vi "Send Voltage.vi"(8 "error in":errorcluster, 11 "69X_79X in":refnum<class "6972A.lvclass">) -> (0 "error out":errorcluster, 3 "69X_79X out":refnum<class "6972A.lvclass">)   [LabVIEW 2019, in "6972A.lvlib" / "6972A.lvclass"]
uses:
  Library/6972A.lvclass
  C:/Users/Public/Documents/Development/builds/Instruments/PowerSupply.lvlibp/Library/PowerSupply.lvclass
  Accessors/Read Local Resource.vi
  Accessors/Write Local Resource.vi
  <instrlib>/Agilent N6900 N7900 Series/Agilent N6900 N7900 Series.lvlib
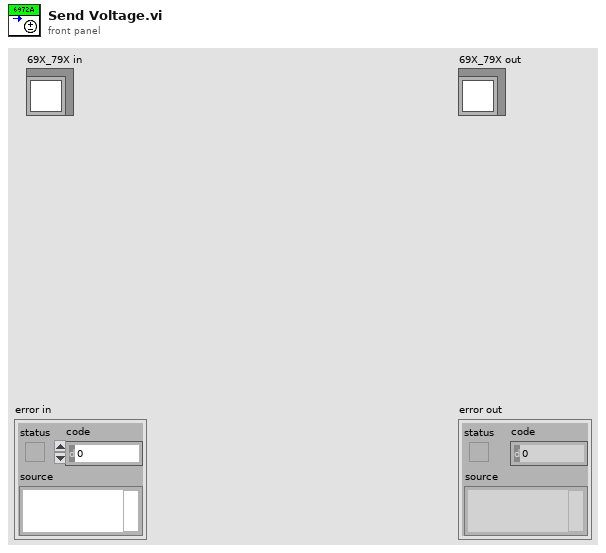
[diagram p1: front panel]
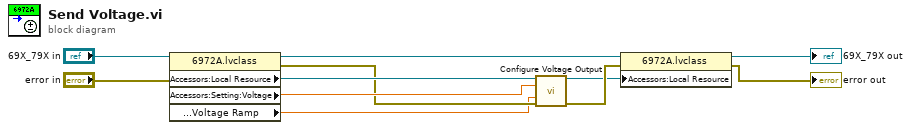
[diagram p0: block diagram]
diagram:
  n1 = property class="6972A.lvclass"(reference="69X_79X in", error in="error in") -> (reference out=w7:refnum<class "6972A.lvclass">, error out=w2:errorcluster, "Accessors:Local Resource"=w3:refnum<visa-resource-name>, "Accessors:Setting:Voltage"=w4:dbl, "Accessors:Setting:Ramp:Voltage Ramp"=w1:dbl)
  n2 = call <instrlib>:"Configure Voltage Output.vi"("VISA resource name"=w3, "Voltage Immediate Amplitude (0 V)"=w4, "Voltage Slew (Inf)"=w1, "error in (no error)"=w2) -> ("VISA resource name out"=w5:refnum<visa-resource-name>, "error out"=w6:errorcluster)  [unwired: 10 in]
  n3 = property class="6972A.lvclass"(reference=w7, error in=w6, "Accessors:Local Resource"=w5) -> (reference out=→"69X_79X out":refnum<class "6972A.lvclass">, error out=→"error out":errorcluster)
